vi "SplashLoader.vi"() -> ()   [LabVIEW 2020]
uses:
  177c2cdc-6276-4d7f-b5d0-e4ff8b7c9410.vi
panel:
  out "URL":string="https://picog.org"
  out "Version":string
  out "Spinner":u8(ring)
  # "Loading picoG Application..."
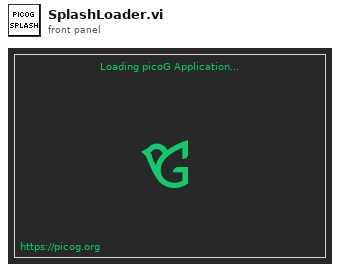
[diagram p1: front panel]
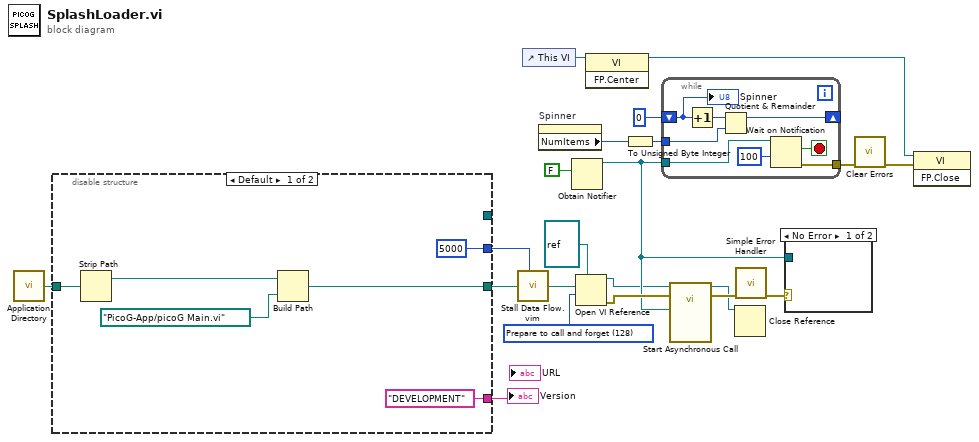
[diagram p0: block diagram]
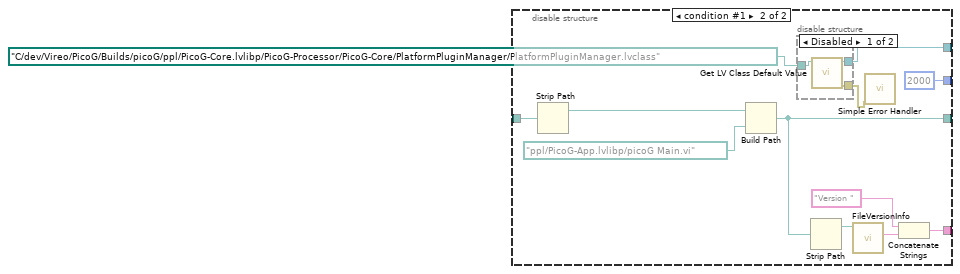
[diagram p2: hidden frame]
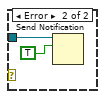
[diagram p4: hidden frame]
diagram:
  w6 = 128 items=["Record modifications"=1, "Open templates for editing"=2, "Prompt user to save"=4, "Prepare for reentrant run"=8, "Prompt to find missing subVIs"=16, "Hide loading dialog box"=32, "Enable simultaneous calls"=64, "Prepare to call and forget"=128, "Simultaneous call and forget"=192, "Prepare to call and collect"=256, "Simultaneous call and collect"=320]
  n1 = call <vilib>:"Application Directory.vi"() -> ("Application Directory"=w12:path)
  n2 = disable-structure shown="Default" {
    disable-tunnel: w12 -> [w27 w31]
    disable-tunnel: [w25 w37] -> w5
    disable-tunnel: ["DEVELOPMENT" ("Version") w33] -> w4
    disable-tunnel: [u32 5000 ("milliseconds to wait") u32 2000 ("milliseconds to wait")] -> w1
    disable-tunnel: [_ w30] -> _
    frame condition #0 (active) {
      n3 = Strip Path(path=w27) -> (stripped path=w26:path)  [unwired: 1 out]
      n4 = Build Path(base path=w26, name or relative path=path "PicoG-App/picoG Main.vi") -> (appended path=w25:path)
    }
    frame condition #1 {
      n5 = Strip Path(path=w31) -> (stripped path=w39:path)  [unwired: 1 out]
      n6 = Build Path(base path=w39, name or relative path=path "ppl/PicoG-App.lvlibp/picoG Main.vi") -> (appended path=w37:path)
      n7 = disable-structure shown="Disabled" {
        disable-tunnel: [w42 _] -> w30
        disable-tunnel: [w41 _] -> w29
        disable-tunnel: path "C:/dev/Vireo/PicoG/Builds/picoG/ppl/PicoG-Core.lvlibp/PicoG-Processor/PicoG-Core/PlatformPluginManager/PlatformPluginManager.lvclass" ("name or relative path") -> [w40 _]
        frame Disabled {
          n8 = call <vilib>:"Get LV Class Default Value.vi"("class path"=w40) -> ("error out"=w41:errorcluster, "object"=w42:refnum<class>)  [unwired: 9 in]
        }
        frame Enabled {
        }
      }
      n9 = Strip Path(path=w37) -> (stripped path=w36:path)  [unwired: 1 out]
      n10 = call <vilib>:"FileVersionInfo.vi"("Application Path in"=w36) -> ("File Version Info"=w35:string)  [unwired: 7 in, 3 out]
      n11 = call <vilib>:"Simple Error Handler.vi"("error in (no error)"=w29) -> ()  [unwired: 4 in, 5 out]
      n12 = Concatenate Strings("Version " ("Version"), w35) -> (w33:string)
    }
  }
  "Version" <- w4
  n13 = call "Stall Data Flow.vim"("value in"=w5, "milliseconds to wait"=w1) -> ("value out"=w2:path)  [unwired: 1 out]
  n14 = control-ref of="This VI"() -> (w19:refnum<vi>)
  n15 = property on="Spinner" class="Ring (strict)"() -> ("NumItems"=w18:u32)  [unwired: 2 in, 2 out]
  n16 = Obtain Notifier(notification data type=FALSE) -> (notifier out=w9:refnum<notifier>)  [unwired: 3 in, 2 out]
  n17 = Open VI Reference(type specifier VI Refnum (for type only)=refnum<vi> refnum, vi path=w2, options=w6) -> (vi reference=w8:refnum<vi>, error out=w10:errorcluster)  [unwired: 3 in]
  n18 = invoke class="VI" method="FP.Center"(reference=w19) -> (reference out=w13:refnum<vi>)  [unwired: 2 in, 2 out]
  n19 = To Unsigned Byte Integer(number=w18) -> (unsigned 8bit integer=w20:u8)
  n20 = while {
    shift-right: [w48] -> _
    shift-left: u8 0 ("Spinner") -> [w50]
    tunnel: w20 -> [w47]
    tunnel: w9 -> [w46]
    tunnel: [w43] -> w15
    stop <- w45 stop-if-true
    n21 = Increment(x=w50) -> (x+1=w49:u8)
    n22 = Quotient & Remainder(x=w49, y=w47) -> (x-y*floor(x/y)=w48:u8)  [unwired: 1 out]
    n23 = Wait on Notification(notifier=w46, timeout in ms (-1)=100) -> (notification=w45:bool, error out=w43:errorcluster)  [unwired: 2 in, 2 out]
    "Spinner" <- w50
  }
  n24 = call-by-ref "Start Asynchronous Call"(reference=w8, error in=w10, "Close Splash Notifier"=w9) -> (reference out=w3:refnum<vi>, error out=w11:errorcluster)  [unwired: 11 in]
  n25 = Close Reference(reference=w3) -> ()  [unwired: 1 in, 1 out]
  n26 = call <vilib>:"Simple Error Handler.vi"("error in (no error)"=w11) -> ("error out"=w16:errorcluster)  [unwired: 4 in, 4 out]
  n27 = case shown="No Error" w16 {
    tunnel: w9 -> [_ w52]
    frame No Error {
    }
    frame Error {
      n28 = Send Notification(notification=TRUE, notifier=w52) -> ()  [unwired: 1 in, 2 out]
    }
  }
  n29 = call <vilib>:"Clear Errors.vi"("error in (no error)"=w15) -> ("error out"=w14:errorcluster)  [unwired: 5 in, 1 out]
  n30 = invoke class="VI" method="FP.Close"(reference=w13, error in=w14) -> ()  [unwired: 1 in, 3 out]
